vi "Units to Scaling Exponent.vi"(3 "Units":string) -> (0 "Scaling Exponent":dbl)   [LabVIEW 2020, in "GUCalibration2.lvlib"]
uses:
  GUCalibration2.lvlib
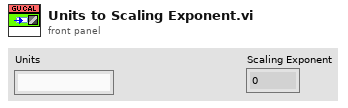
[diagram p1: front panel]
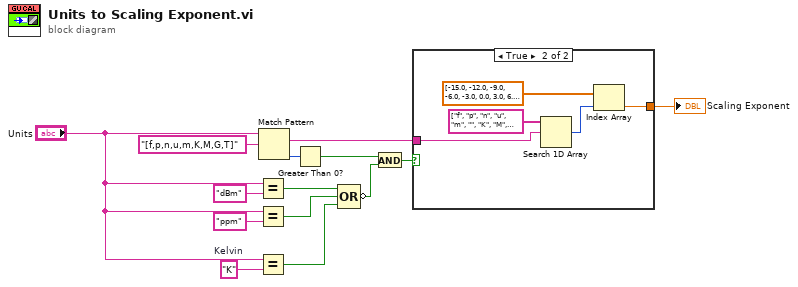
[diagram p0: block diagram]
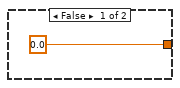
[diagram p2: hidden frame]
diagram:
  w6 = "K"  # Kelvin
  n1 = Equal?(x="Units", y="dBm" ("spreadsheet string 2")) -> (x = y?=w4:bool)
  n2 = Equal?(x="Units", y="ppm") -> (x = y?=w3:bool)
  n3 = Equal?(x="Units", y=w6) -> (x = y?=w8:bool)
  n4 = Match Pattern(string="Units", regular expression="[f,p,n,u,m,K,M,G,T]" ("spreadsheet string 2")) -> (match substring=w12:string, offset past match=w13:i32)  [unwired: 1 in, 2 out]
  n5 = Greater Than 0?(x=w13) -> (x > 0?=w9:bool)
  n6 = Compound Arithmetic op=OR(w4, w3, w8) -> (invert w7:bool)
  n7 = And(x=w9, y=w7) -> (x .and. y?=w10:bool)
  n8 = case shown="True" w10 {
    tunnel: w12 -> [_ w20]
    tunnel: [0.0 w18] -> w11
    frame False {
    }
    frame True {
      n9 = Search 1D Array(1D array=string[] ["f", "p", "n", "u", "m", "", "K", "M", "G", "T"] ("Strings []"), element=w20) -> (index of element=w19:i32)  [unwired: 1 in]
      n10 = Index Array(array=dbl[] [-15.0, -12.0, -9.0, -6.0, -3.0, 0.0, 3.0, 6.0, 9.0, 12.0] ("Strings []"), index=w19) -> (element=w18:dbl)
    }
  }
  "Scaling Exponent" <- w11
